vi "light_sensor.vi"() -> ()   [LabVIEW 2018]
uses:
  <vilib>/DAQmx/read.llb/DAQmx Read (Analog DBL 1Chan 1Samp).vi
  <vilib>/DAQmx/miscellaneous.llb/DAQmx Fill In Error Info.vi
panel:
  out "err out":refnum<k21>
  out "Meter":dbl(knob) scale=0.0..20.0
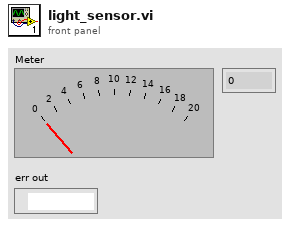
[diagram p1: front panel]
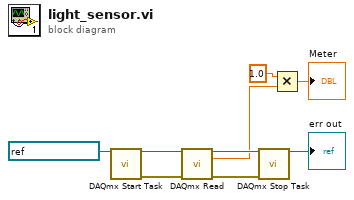
[diagram p0: block diagram]
diagram:
  n1 = call <vilib>:"DAQmx Start Task.vi"("task/channels in"=refnum<k21> "light_sensor") -> ("task out"=w6:refnum<k21>, "error out"=w8:errorcluster)  [unwired: 13 in]
  n2 = call-poly <vilib>:"DAQmx Read.vi"("task/channels in"=w6, "error in"=w8) -> ("task out"=w7:refnum<k21>, "data"=w4:dbl, "error out"=w9:errorcluster)  [unwired: 11 in]
  n3 = call <vilib>:"DAQmx Stop Task.vi"("task/channels in"=w7, "error in"=w9) -> ("task out"=→"err out":refnum<k21>)  [unwired: 12 in, 1 out]
  n4 = Multiply(x=1.0, y=w4) -> (x*y=→"Meter":dbl)
